vi "FlexRay_Demo.vi"() -> ()   [LabVIEW 2023]
uses:
  <vilib>/Utility/error.llb/Trim Whitespace One-Sided.vi
  D:/LabVIEW/TSMaster_FlexRay_Labview/Interop.TSMasterAPI.dll
  Interop.TSMasterAPI.dll
panel:
  in  "Refresh":bool
  in  "EnableReceive":bool
  in  "FlexRayFrame":i32(listbox) caption="报文显示"
  in  "Transmit":bool
  in  "Array":u8[](array[numeric])=[1, 2, 3, 4, 5, 6, 7, 8, 9, 10, 11] format="%.0x"
  in  "Connect":bool
  in  "HardwareConfig":bool
  in  "Exit":bool
  in  "LoadProject":bool
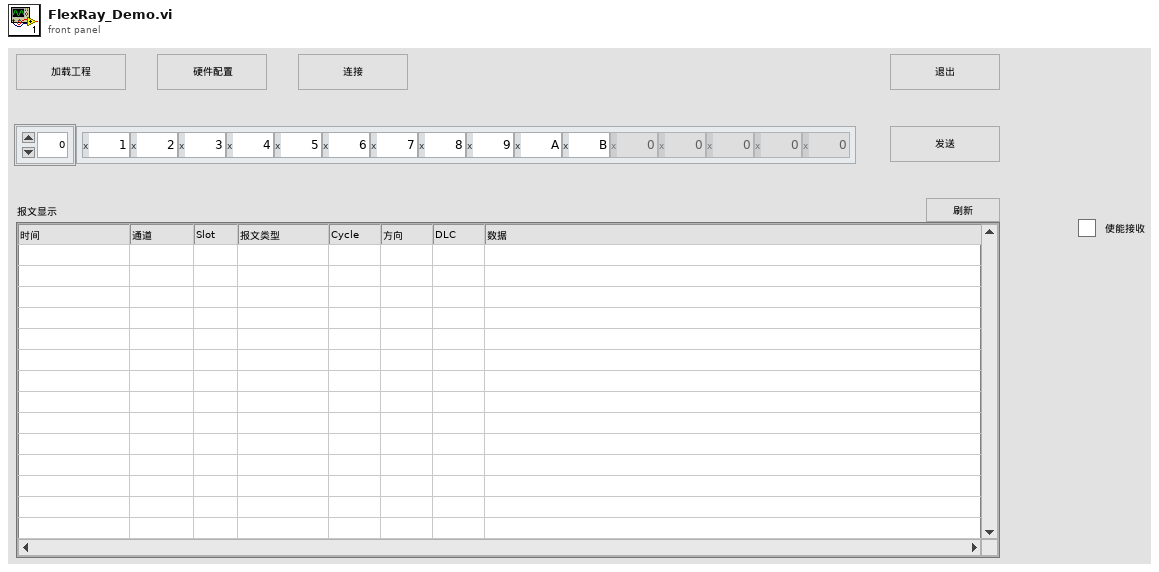
[diagram p1: front panel]
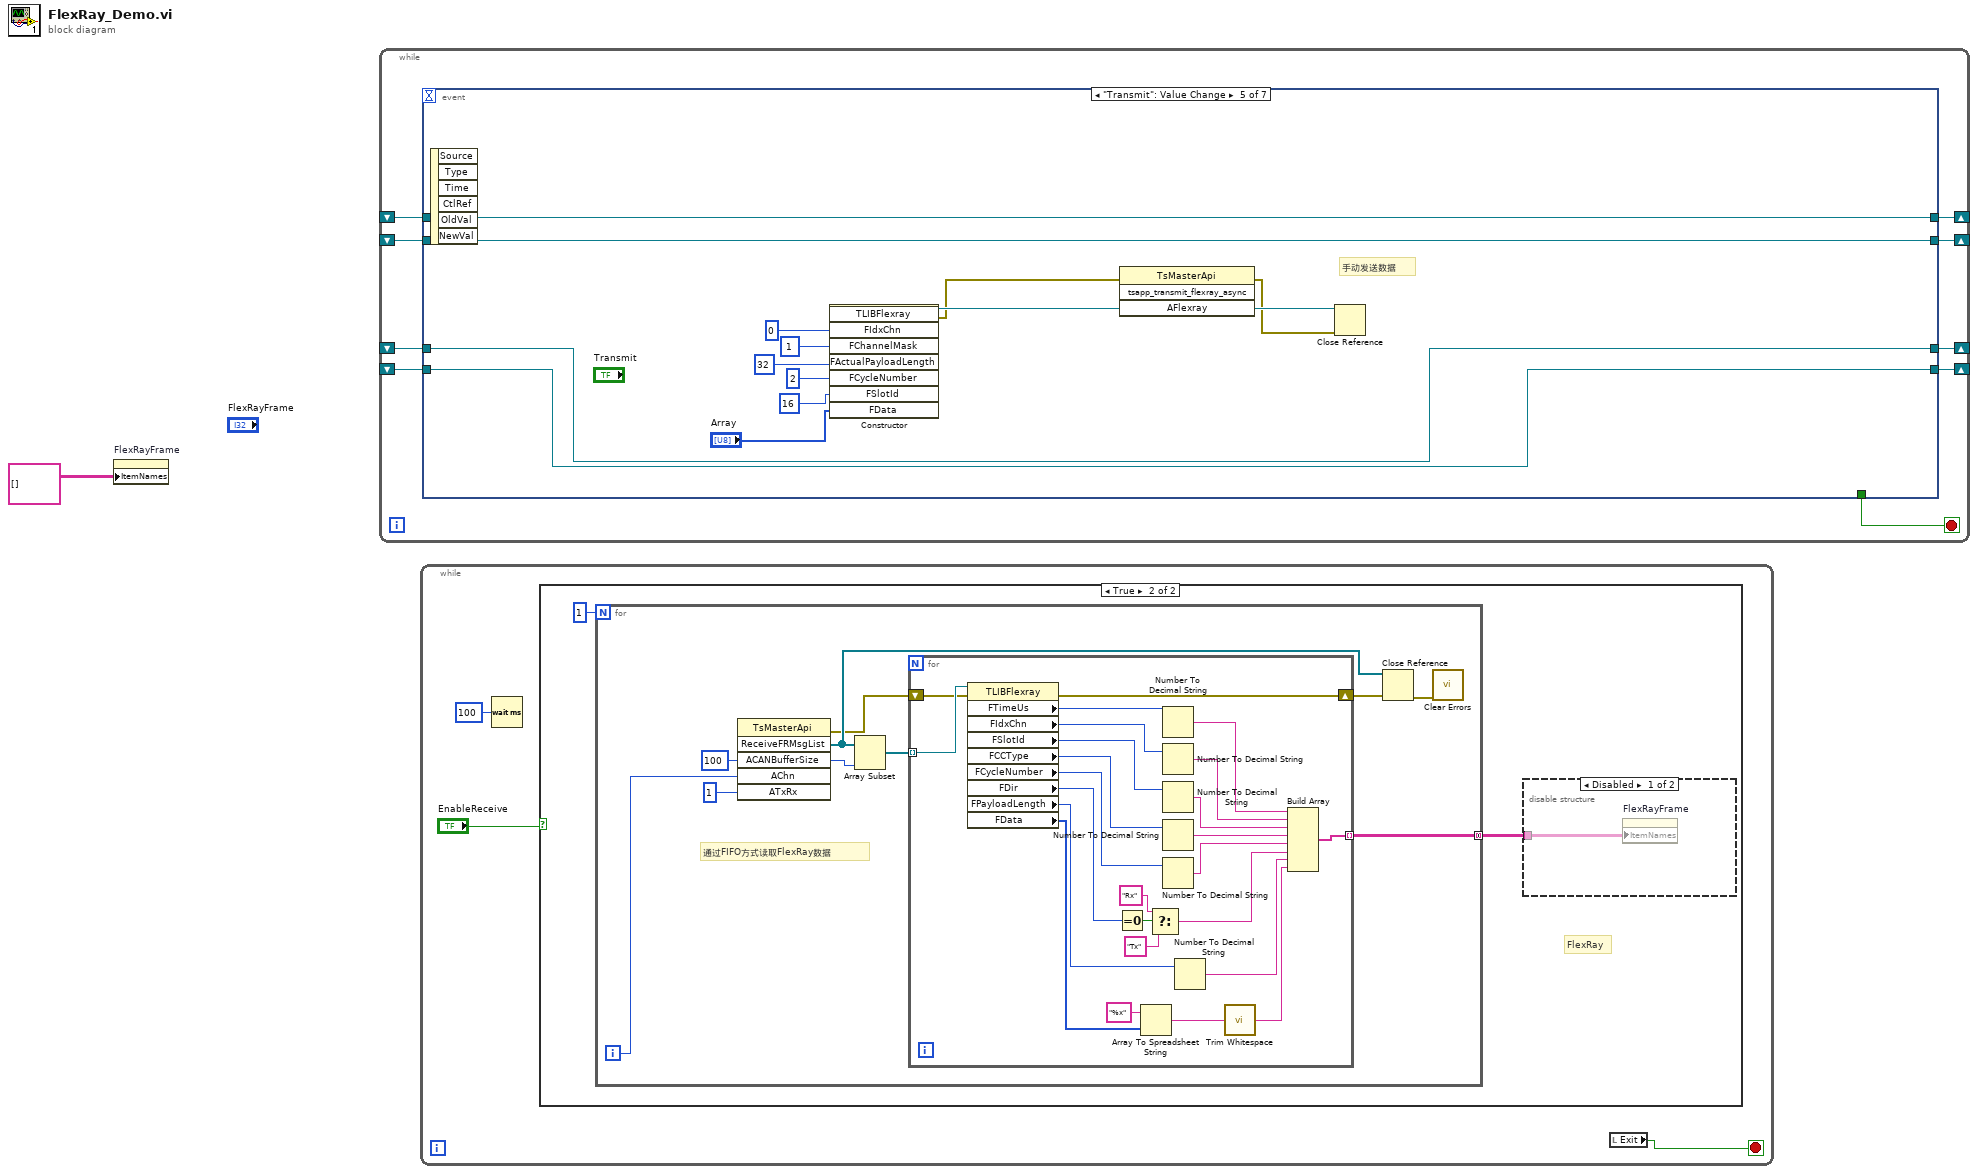
[diagram p0: block diagram]
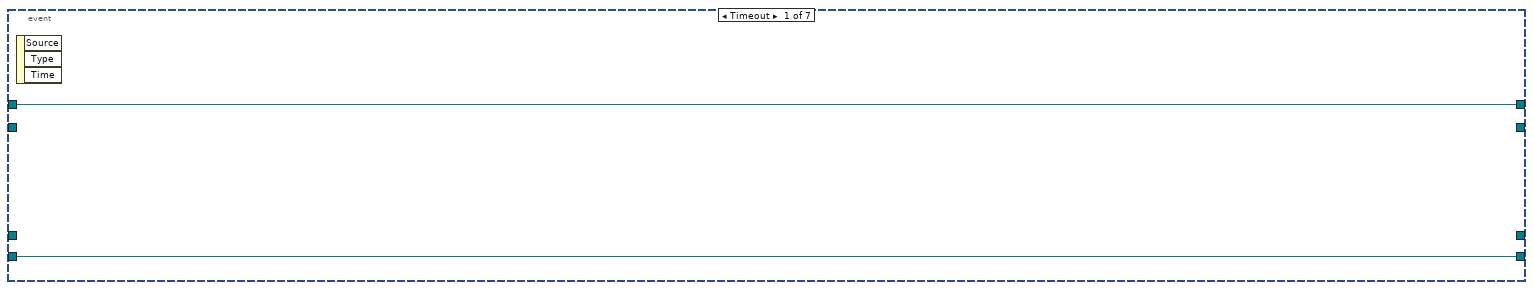
[diagram p4: hidden frame]
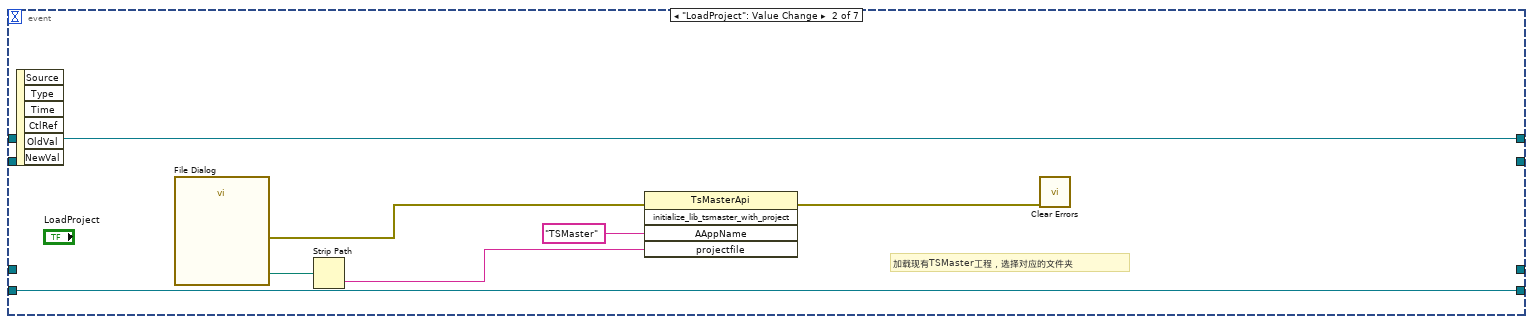
[diagram p5: hidden frame]
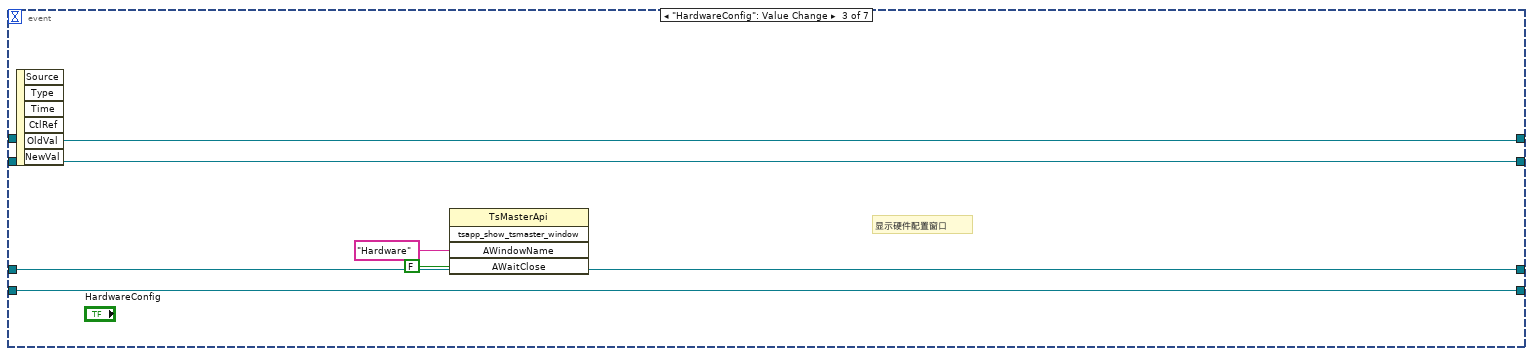
[diagram p6: hidden frame]
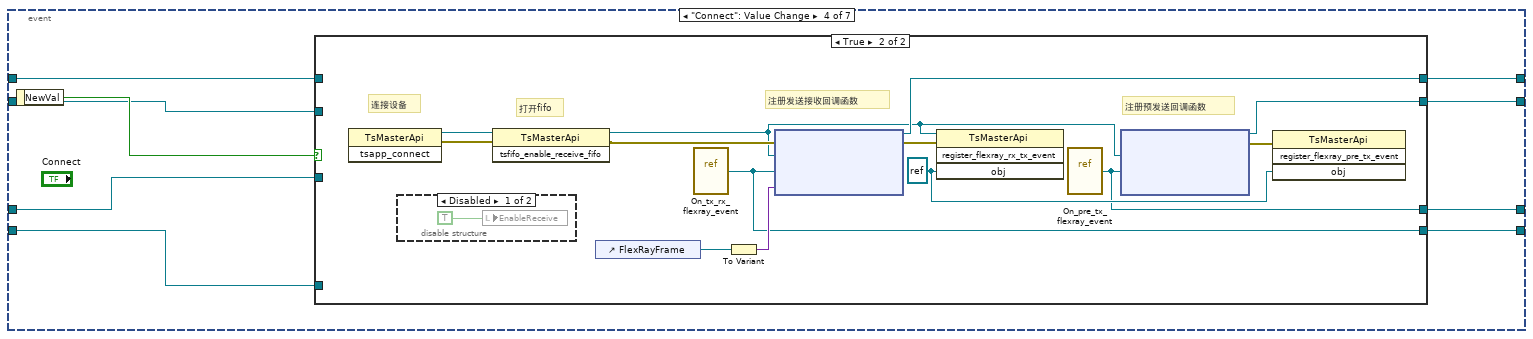
[diagram p7: hidden frame]
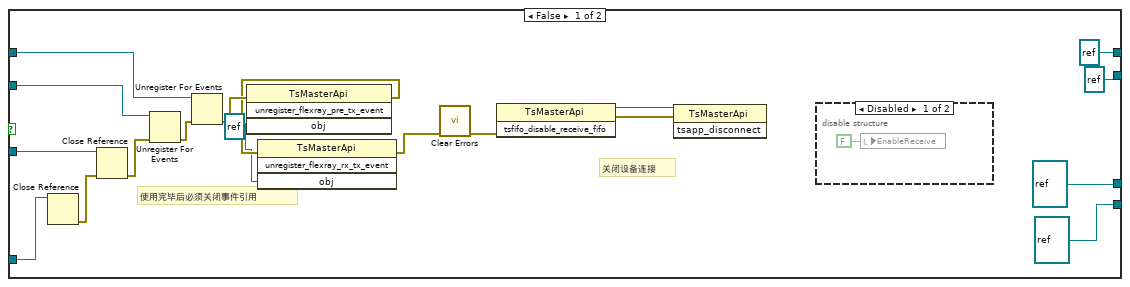
[diagram p8: hidden frame]
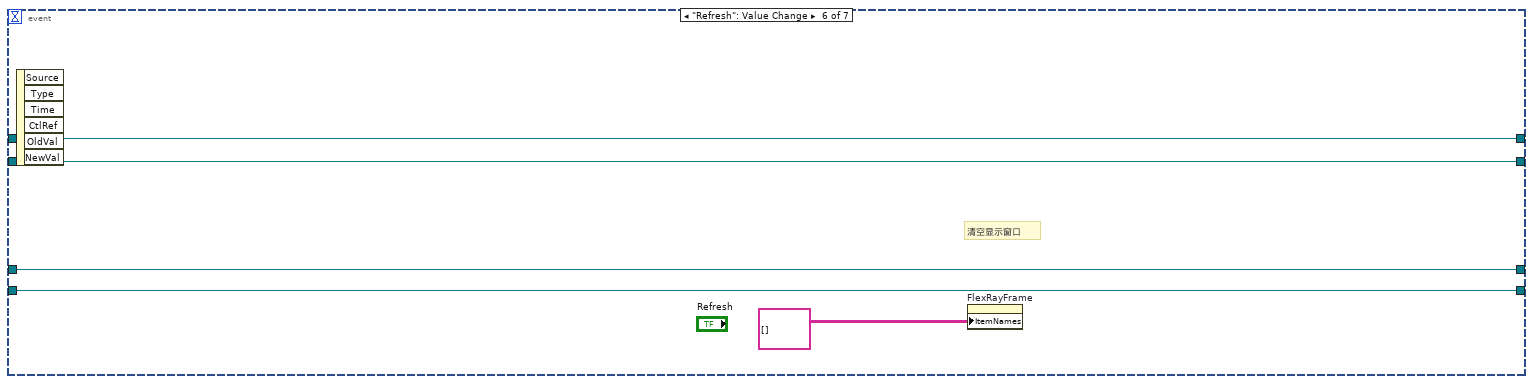
[diagram p11: hidden frame]
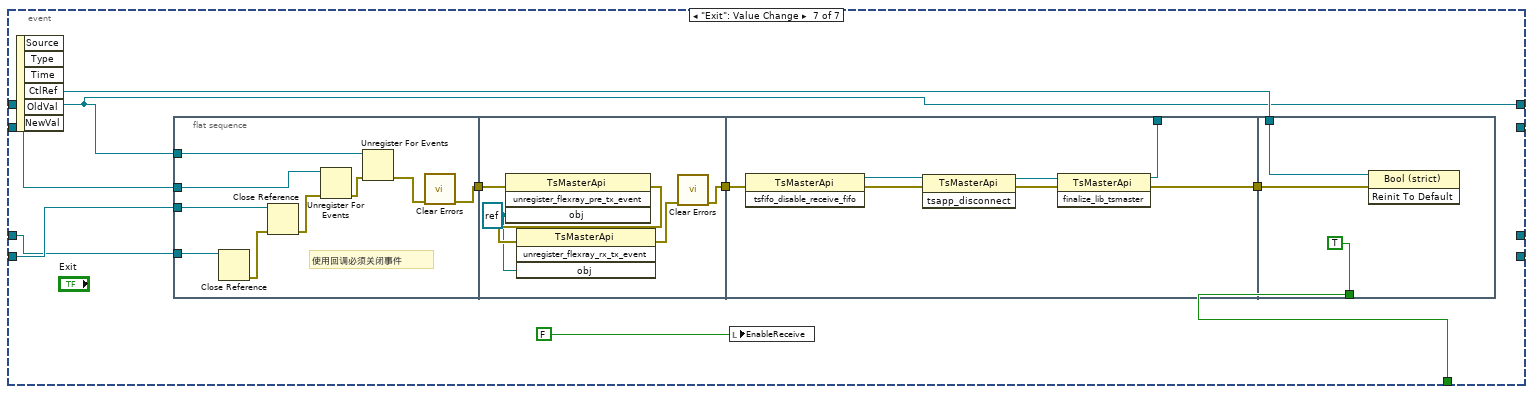
[diagram p12: hidden frame]
diagram:
  n1 = property on="FlexRayFrame" class="MCListbox (strict)"("ItemNames"=string[][] [] ("Item Names")) -> ()  [unwired: 2 in, 2 out]
  n2 = while {
    shift-right: [w9] -> _
    shift-left: _ -> [w8]
    shift-right: [w7] -> _
    shift-left: _ -> [w6]
    shift-right: [w5] -> _
    shift-left: _ -> [w3]
    shift-right: [w4] -> _
    shift-left: _ -> [w2]
    stop <- w10 stop-if-true
    n3 = event shown="[4] \"Transmit\": Value Change" {
      selector: _ -> [_ _ _ _ _ _ _]
      dyn-events: _ -> [_ _ _ _ _ _ _]
      timeout: _ -> [_ _ _ _ _ _ _]
      tunnel: [_ _ _ _ _ _ w94] -> w10
      tunnel: [w12 w14 w23 w33 w71 w86 w92] -> w9
      tunnel: w8 -> [w12 w14 w23 w32 w71 w86 w92]
      tunnel: [w11 w13 w22 w31 w70 w83 _] -> w7
      tunnel: w6 -> [w11 w13 w22 w30 w70 w83 w91]
      tunnel: [_ _ w21 w29 w69 w85 _] -> w5
      tunnel: [_ _ w20 w28 w68 w84 _] -> w4
      tunnel: w3 -> [_ _ w21 w26 w69 w85 w90]
      tunnel: w2 -> [_ _ w20 w27 w68 w84 w89]
      event Timeout {
        n4 = event-data() -> ()  [unwired: 1 in, 3 out]
      }
      event "LoadProject": Value Change {
        # "加载现有TSMaster工程，选择对应的文件夹"
        n5 = event-data() -> ()  [unwired: 1 in, 6 out]
        n6 = call "File Dialog"() -> ("selected path"=w19:path, "error out"=w16:errorcluster)  [unwired: 12 in, 2 out]
        n7 = Strip Path(path=w19) -> (name=w18:string)  [unwired: 1 out]
        n8 = invoke class="TsMasterApi" method="initialize_lib_tsmaster_with_project"(error in=w16, "AAppName"="TSMaster", "projectfile"=w18) -> (error out=w17:errorcluster)  [unwired: 2 in, 4 out]
        n9 = call <vilib>:"Clear Errors.vi"("error in (no error)"=w17) -> ()  [unwired: 5 in, 2 out]
      }
      event "HardwareConfig": Value Change {
        # "显示硬件配置窗口"
        n10 = event-data() -> ()  [unwired: 1 in, 6 out]
        n11 = invoke class="TsMasterApi" method="tsapp_show_tsmaster_window"("AWindowName"="Hardware", "AWaitClose"=FALSE) -> ()  [unwired: 3 in, 5 out]
      }
      event "Connect": Value Change {
        n12 = event-data() -> ("NewVal"=w34:bool)  [unwired: 1 in]
        n13 = case shown="True" w34 {
          tunnel: [refnum<k27> refnum ("Event Callback") w60] -> w33
          tunnel: w32 -> [w49 _]
          tunnel: [refnum<vi> refnum ("vi reference") w59] -> w31
          tunnel: w30 -> [w50 _]
          tunnel: [refnum<k27> refnum ("Event Callback") w56] -> w29
          tunnel: [refnum<vi> refnum ("vi reference") w55] -> w28
          tunnel: w27 -> [w44 _]
          tunnel: w26 -> [w42 _]
          frame False {
            w35 = refnum<k24> refnum ("obj")
            # "关闭设备连接"
            # "使用完毕后必须关闭事件引用"
            n14 = Close Reference(reference=w50) -> (error out=w43:errorcluster)  [unwired: 1 in]
            n15 = Close Reference(reference=w44, error in (no error)=w43) -> (error out=w41:errorcluster)
            n16 = Unregister For Events(event registration refnum=w42, error in=w41) -> (error out=w40:errorcluster)
            n17 = Unregister For Events(event registration refnum=w49, error in=w40) -> (error out=w38:errorcluster)
            n18 = invoke class="TsMasterApi" method="unregister_flexray_pre_tx_event"(error in=w38, "obj"=w35) -> (error out=w37:errorcluster)  [unwired: 2 in, 3 out]
            n19 = invoke class="TsMasterApi" method="unregister_flexray_rx_tx_event"(error in=w37, "obj"=w35) -> (error out=w36:errorcluster)  [unwired: 2 in, 3 out]
            n20 = call <vilib>:"Clear Errors.vi"("error in (no error)"=w36) -> ("error out"=w39:errorcluster)  [unwired: 5 in, 1 out]
            n21 = invoke class="TsMasterApi" method="tsfifo_disable_receive_fifo"(error in=w39) -> (reference out=w51:refnum<k24>, error out=w52:errorcluster)  [unwired: 2 in, 1 out]
            n22 = invoke class="TsMasterApi" method="tsapp_disconnect"(reference=w51, error in=w52) -> ()  [unwired: 1 in, 3 out]
            n23 = disable-structure shown="Disabled" {
              frame Disabled {
                n24 = local write "EnableReceive"(FALSE ("EnableReceive")) -> ()
              }
              frame Enabled {
              }
            }
          }
          frame True {
            w57 = refnum<k24> refnum ("obj")
            # "注册预发送回调函数"
            # "注册发送接收回调函数"
            # "打开fifo"
            # "连接设备"
            n25 = invoke class="TsMasterApi" method="tsapp_connect"() -> (reference out=w61:refnum<k24>, error out=w66:errorcluster)  [unwired: 3 in, 1 out]
            n26 = disable-structure shown="Disabled" {
              frame Disabled {
                n27 = local write "EnableReceive"(TRUE ("EnableReceive")) -> ()
              }
              frame Enabled {
              }
            }
            n28 = invoke class="TsMasterApi" method="tsfifo_enable_receive_fifo"(reference=w61, error in=w66) -> (reference out=w58:refnum<k24>, error out=w63:errorcluster)  [unwired: 1 in, 1 out]
            n29 = control-ref of="FlexRayFrame"() -> (w62:refnum<vi>)
            n30 = vi-ref "On_tx_rx_flexray_event.vi"() -> ("vi reference"=w59:refnum<vi>)
            n31 = To Variant(anything=w62) -> (Variant=w65:variant)
            n32 = node(w63, w58, w59, w65) -> (w60:refnum<k27>, w64:errorcluster)  [unwired: 1 in]
            n33 = invoke class="TsMasterApi" method="register_flexray_rx_tx_event"(reference=w58, error in=w64, "obj"=w57) -> ()  [unwired: 1 in, 4 out]
            n34 = vi-ref "On_pre_tx_flexray_event.vi"() -> ("vi reference"=w55:refnum<vi>)
            n35 = node(w58, w55) -> (w56:refnum<k27>, w54:errorcluster)  [unwired: 3 in]
            n36 = invoke class="TsMasterApi" method="register_flexray_pre_tx_event"(error in=w54, "obj"=w57) -> ()  [unwired: 2 in, 4 out]
          }
        }
      }
      event "Transmit": Value Change {
        # "手动发送数据"
        n37 = event-data() -> ()  [unwired: 1 in, 6 out]
        n38 = constructor class="TLIBFlexray"("FIdxChn"=u8 0, "FChannelMask"=u8 1, "FActualPayloadLength"=u8 32, "FCycleNumber"=u8 2, "FSlotId"=u16 16, "FData"="Array") -> (reference out=w75:refnum<k24>, error out=w73:errorcluster)  [unwired: 3 in, 7 out]
        n39 = invoke class="TsMasterApi" method="tsapp_transmit_flexray_async"(error in=w73, "AFlexray"=w75) -> (error out=w72:errorcluster, "AFlexray"=w74:refnum<k24>)  [unwired: 2 in, 2 out]
        n40 = Close Reference(reference=w74, error in (no error)=w72) -> ()  [unwired: 1 out]
      }
      event "Refresh": Value Change {
        # "清空显示窗口"
        n41 = event-data() -> ()  [unwired: 1 in, 6 out]
        n42 = property on="FlexRayFrame" class="MCListbox (strict)"("ItemNames"=string[][] [] ("Item Names")) -> ()  [unwired: 2 in, 2 out]
      }
      event "Exit": Value Change {
        n43 = event-data() -> ("CtlRef"=w96:refnum<vi>)  [unwired: 1 in, 5 out]
        n44 = flat-sequence {
          tunnel: w92 -> [w101]
          tunnel: w91 -> [w99]
          tunnel: [w105] -> w88
          tunnel: w90 -> [w100]
          tunnel: w89 -> [w98]
          tunnel: w88 -> [w110]
          tunnel: [w106] -> w87
          tunnel: [w114] -> w95
          tunnel: [w112] -> _
          tunnel: w87 -> [w111]
          tunnel: w96 -> [w120]
          tunnel: w95 -> [w119]
          tunnel: [TRUE] -> w94
          frame #0 {
            # "使用回调必须关闭事件"
            n45 = Close Reference(reference=w98) -> (error out=w104:errorcluster)  [unwired: 1 in]
            n46 = Close Reference(reference=w99, error in (no error)=w104) -> (error out=w103:errorcluster)
            n47 = Unregister For Events(event registration refnum=w100, error in=w103) -> (error out=w102:errorcluster)
            n48 = Unregister For Events(event registration refnum=w101, error in=w102) -> (error out=w97:errorcluster)
            n49 = call <vilib>:"Clear Errors.vi"("error in (no error)"=w97) -> ("error out"=w105:errorcluster)  [unwired: 5 in, 1 out]
          }
          frame #1 {
            w108 = refnum<k24> refnum ("obj")
            n50 = invoke class="TsMasterApi" method="unregister_flexray_pre_tx_event"(error in=w110, "obj"=w108) -> (error out=w109:errorcluster)  [unwired: 2 in, 3 out]
            n51 = invoke class="TsMasterApi" method="unregister_flexray_rx_tx_event"(error in=w109, "obj"=w108) -> (error out=w107:errorcluster)  [unwired: 2 in, 3 out]
            n52 = call <vilib>:"Clear Errors.vi"("error in (no error)"=w107) -> ("error out"=w106:errorcluster)  [unwired: 5 in, 1 out]
          }
          frame #2 {
            n53 = invoke class="TsMasterApi" method="tsfifo_disable_receive_fifo"(error in=w111) -> (reference out=w113:refnum<k24>, error out=w117:errorcluster)  [unwired: 2 in, 1 out]
            n54 = invoke class="TsMasterApi" method="tsapp_disconnect"(reference=w113, error in=w117) -> (reference out=w116:refnum<k24>, error out=w115:errorcluster)  [unwired: 1 in, 1 out]
            n55 = invoke class="TsMasterApi" method="finalize_lib_tsmaster"(reference=w116, error in=w115) -> (reference out=w112:refnum<k24>, error out=w114:errorcluster)  [unwired: 1 in, 1 out]
          }
          frame #3 {
            n56 = invoke class="Bool (strict)" method="Reinit To Default"(reference=w120, error in=w119) -> ()  [unwired: 1 in, 3 out]
          }
        }
        n57 = local write "EnableReceive"(FALSE ("EnableReceive")) -> ()
      }
    }
  }
  n58 = while {
    stop <- w121 stop-if-true
    n59 = Wait (ms)(milliseconds to wait=u32 100) -> ()  [unwired: 1 out]
    n60 = case shown="True" "EnableReceive" {
      frame False {
      }
      frame True {
        # "FlexRay"
        n61 = for {
          N: 1 -> [_]
          tunnel: [w131] -> w124 mode=concatenating
          i -> [w136]
          # "通过FIFO方式读取FlexRay数据"
          n62 = invoke class="TsMasterApi" method="ReceiveFRMsgList"("ACANBufferSize"=100, "AChn"=w136, "ATxRx"=u8 1) -> (error out=w129:errorcluster, "ReceiveFRMsgList"=w130:refnum<k24>[], "ACANBufferSize"=w133:i32)  [unwired: 3 in, 3 out]
          n63 = Array Subset(array=w130, length=w133) -> (w132:refnum<k24>[])  [unwired: 1 in]
          n64 = for {
            tunnel: w132 -> [w161] mode=indexing
            tunnel: [w142] -> w131 mode=indexing
            shift-right: [w140] -> w128
            shift-left: w129 -> [w141]
            n65 = property class="TLIBFlexray"(reference=w161, error in=w141) -> (error out=w140:errorcluster, "FTimeUs"=w160:u64, "FIdxChn"=w159:u8, "FSlotId"=w158:u16, "FCCType"=w150:u8, "FCycleNumber"=w157:u8, "FDir"=w155:u8, "FPayloadLength"=w139:u8, "FData"=w152:u8[])  [unwired: 1 out]
            n66 = Equal To 0?(x=w155) -> (x = 0?=w156:bool)
            n67 = Array To Spreadsheet String(array=w152, 3:"%x" ("format string")) -> (spreadsheet string=w143:string)  [unwired: 1 in]
            n68 = Select(t="Rx", s=w156, f="Tx") -> (s? t:f=w144:string)
            n69 = Number To Decimal String(number=w160) -> (decimal integer string=w149:string)  [unwired: 1 in]
            n70 = Number To Decimal String(number=w159) -> (decimal integer string=w148:string)  [unwired: 1 in]
            n71 = Number To Decimal String(number=w158) -> (decimal integer string=w147:string)  [unwired: 1 in]
            n72 = Number To Decimal String(number=w150) -> (decimal integer string=w146:string)  [unwired: 1 in]
            n73 = Number To Decimal String(number=w157) -> (decimal integer string=w145:string)  [unwired: 1 in]
            n74 = Number To Decimal String(number=w139) -> (decimal integer string=w138:string)  [unwired: 1 in]
            n75 = call <vilib>:"Trim Whitespace.vi"("string"=w143) -> ("trimmed string"=w137:string)  [unwired: 1 in]
            n76 = Build Array(w149, w148, w147, w146, w145, w144, w138, w137) -> (w142:string[])
          }
          n77 = Close Reference(reference=w130, error in (no error)=w128) -> (error out=w127:errorcluster)
          n78 = call <vilib>:"Clear Errors.vi"("error in (no error)"=w127) -> ()  [unwired: 5 in, 2 out]
        }
        n79 = disable-structure shown="Disabled" {
          disable-tunnel: w124 -> [w126 _]
          frame Disabled {
            n80 = property on="FlexRayFrame" class="MCListbox (strict)"("ItemNames"=w126) -> ()  [unwired: 2 in, 2 out]
          }
          frame Enabled {
          }
        }
      }
    }
    n81 = local read "Exit"() -> (w121:bool)
  }
